vi "Error Add To Que.vi"(11 "Error Code":i32=5000) -> ()   [LabVIEW 2019]
uses:
  LLB/Message/Ctrl/MsgDataInput.ctl
  LLB/Message/Ctrl/MsgPageSelect.ctl
  LLB/Message/Ctrl/LogType.ctl
  Ctrl/AlarmReportCtrl.ctl
  LLB/Commonly VI/Main Glb.vi
  LLB/Message/MsgShowAndLog.lvlib
  LLB/Commonly VI.lvlib
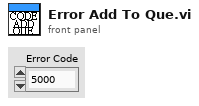
[diagram p1: front panel]
types:
  T1 = typedef "AlarmReportCtrl.ctl" = enum16{"Initial", "AddError", "WriteAlarmResetTime", "WriteOPID", "Load", "Save", "WriteRootCause"}
  T2 = typedef "MsgDataInput.ctl" = cluster{"MsgPageSelect":T3, "LogType":T4, "Msg":string, "Time":string}
  T3 = typedef "MsgShowAndLog.lvlib/MsgPageSelect.ctl" = enum16{"System", "Comm", "IO", "Action", "Alarm"}
  T4 = typedef "MsgShowAndLog.lvlib/LogType.ctl" = enum16{"Auto", "Manual", "Handshake", "Error"}
  T5 = cluster{"status":bool, "Error Code":i32, "String":string}
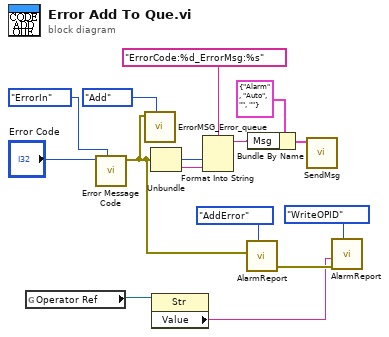
[diagram p0: block diagram]
diagram:
  n1 = global read "Main Glb.vi" "Operator Ref"() -> (w2:refnum<vi>)
  n2 = call "Error Message Code.vi"("Enum"=enum16{"Initial", "ErrorIn"}."ErrorIn", "Error Code"="Error Code") -> ("Error Message"=w5:T5)  [unwired: 9 in]
  n3 = call "ErrorMSG_Error_queue.vi"("Method"=enum16{"Initial", "Add", "Read", "Delete"}."Add", "queue element"=w5) -> ()  [unwired: 7 in, 3 out]
  n4 = Unbundle(w5) -> ("Error Code"=w10:i32, "String"=w9:string)  [unwired: 1 out]
  n5 = property class="Str"(reference=w2) -> ("Value"=w1:string)  [unwired: 1 in, 2 out]
  n6 = Format Into String(format string="ErrorCode:%d_ErrorMsg:%s", w10, w9) -> (resulting string=w12:string)  [unwired: 2 in, 1 out]
  n7 = call "AlarmReport.vi"("Emun"=AlarmReportCtrl."AddError", "error In"=w5) -> ("error out"=w3:errorcluster)  [unwired: 9 in]
  n8 = Bundle By Name(cluster=T2 {"MsgPageSelect"=enum."Alarm", "LogType"=enum."Auto", "Msg"="", "Time"=""} ("DataIn"), "Msg"=w12) -> (w8:T2)
  n9 = call "SendMsg.vi"("DataIn"=w8) -> ()  [unwired: 10 in, 1 out]
  n10 = call "AlarmReport.vi"("Emun"=AlarmReportCtrl."WriteOPID", "VILinkerror In"=w3, "OPID"=w1) -> ()  [unwired: 8 in, 1 out]
